vi "Process Data PID 0 Set_vel.vi"(0 "A_Pos":i32, 1 "Target Pos Set":i32, 5 "dt IN (s)":dbl=-1.0 format="%.8f", 8 "Num":i32, 10 "PID Set Time(ms)":i32, 11 "output range":cluster{"output high":dbl, "output low":dbl}={"output high"=100.0, "output low"=-100.0} caption="Velo Limd" {"output low" format="%.2f"; "output high" format="%.2f"}, 13 "PID gains":T1={"proportional gain (Kc)"=1.0, "integral time (Ti, min)"=0.01, "derivative time (Td, min)"=0.0} caption="Pos PID Gain" {"derivative time (Td, min)" format="%.7f"; "integral time (Ti, min)" format="%.7f"; "proportional gain (Kc)" format="%.7f"}) -> (14 "output":i32 caption="OUTPUT", 15 "Target Pos":i32, 19 "dt OUT (s)":dbl format="%.8f")   [LabVIEW 2019]
uses:
  <vilib>/addons/control/pid/pid.llb/PID (DBL).vi
  <vilib>/addons/control/pid/NI_PID_pid.lvlib
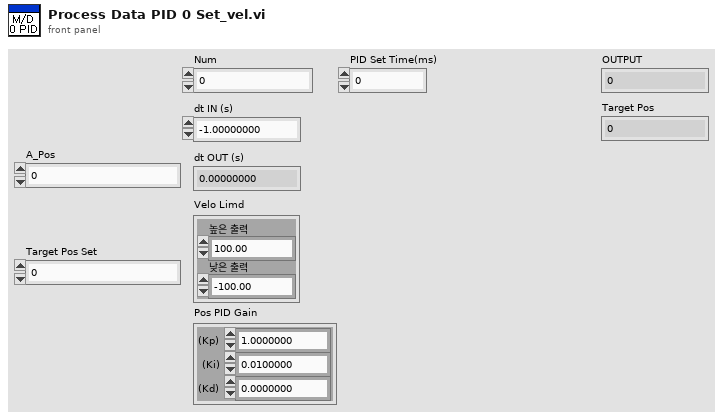
[diagram p1: front panel]
types:
  T1 = cluster{"proportional gain (Kc)":dbl, "integral time (Ti, min)":dbl, "derivative time (Td, min)":dbl}
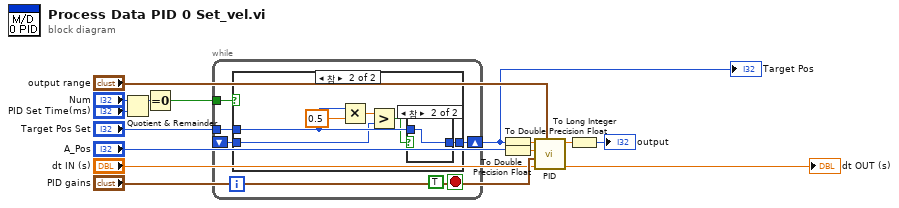
[diagram p0: block diagram]
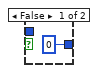
[diagram p3: hidden frame]
diagram:
  n1 = Quotient & Remainder(x="Num", y="PID Set Time(ms)") -> (x-y*floor(x/y)=w8:i32)  [unwired: 1 out]
  n2 = Equal To 0?(x=w8) -> (x = 0?=w10:bool)
  n3 = while {
    tunnel: w10 -> [w20]
    shift-right: [w19] -> w6
    shift-left: _ -> [w17]
    tunnel: "Target Pos Set" -> [w16]
    stop <- TRUE stop-if-true
    n4 = case shown="참" w20 {
      tunnel: w16 -> [_ w26]
      tunnel: w17 -> [w21 w23]
      tunnel: [w21 w27] -> w19
      frame False {
      }
      frame True {
        n5 = Multiply(x=w26, y=sgl 0.5) -> (x*y=w24:sgl)
        n6 = Greater?(x=w24, y=w23) -> (0:w22:bool)
        n7 = case shown="참" w22 {
          tunnel: w26 -> [_ w29]
          tunnel: [0 ("Target Pos Set") w29] -> w27
          frame False {
          }
          frame True {
          }
        }
      }
    }
  }
  "Target Pos" <- w6
  n8 = To Double Precision Float(number=w6) -> (double precision float=w4:dbl)
  n9 = To Double Precision Float(number="A_Pos") -> (double precision float=w3:dbl)
  n10 = call-poly <vilib>:"PID.vi"("output range"="output range", "dt (s)"="dt IN (s)", "PID gains"="PID gains", "process variable"=w3, "setpoint"=w4) -> ("dt out (s)"=→"dt OUT (s)":dbl, "output"=w1:dbl)  [unwired: 5 in]
  n11 = To Long Integer(number=w1) -> (32bit integer=→"output":i32)
